vi "Generate Thetas.vi"(0 "spline flat":cluster{"x":sgl, "y":sgl}[](array[cluster]), 5 "starting angle":sgl, 7 "dt":sgl=0.02, 9 "ctrl pts":cluster{sgl, sgl}[][](array[cluster]), 11 "y unflat":cluster{dbl[]}[](array[cluster])) -> (4 "omega":sgl[](array[numeric]), 6 "theta":sgl[](array[numeric]), 10 "Tangent Vector":cluster{"x out":dbl, "y out":dbl}[](array[cluster]))   [LabVIEW 2025]
uses:
  <vilib>/Analysis/NI_AALPro.lvlib
panel:
  out "error":i32
  out "integral of P(x)":dbl
  out "Better omega":dbl(graph)
  out "Omega Theta":cluster{sgl, sgl}(graph)
  out "Array 2":sgl[](array[numeric])
  out "Array":sgl[](array[numeric])
  out "Thetas":sgl(graph)
  out "Omegas":sgl(graph)
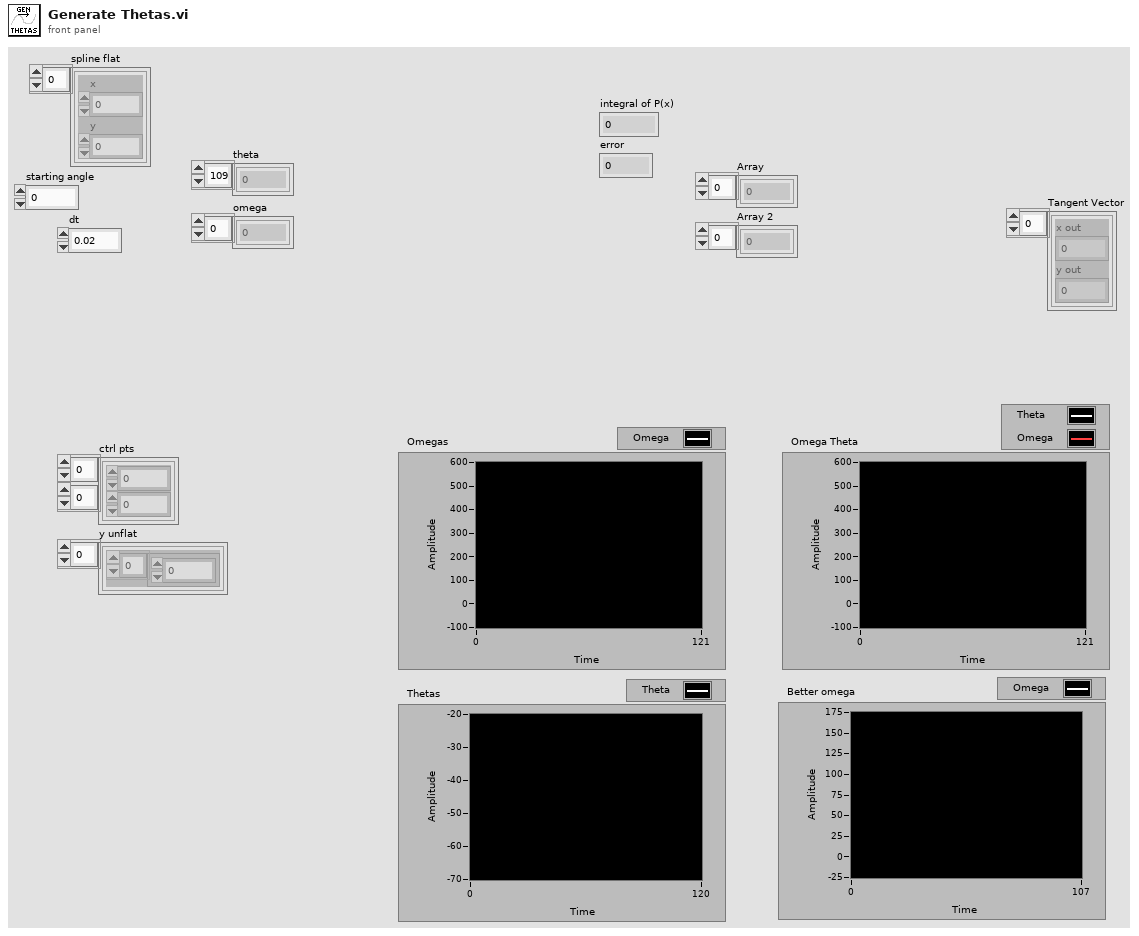
[diagram p1: front panel]
types:
  T1 = typedef "Bezier Curve.ctl" = cluster{"x":sgl, "y":sgl}[]
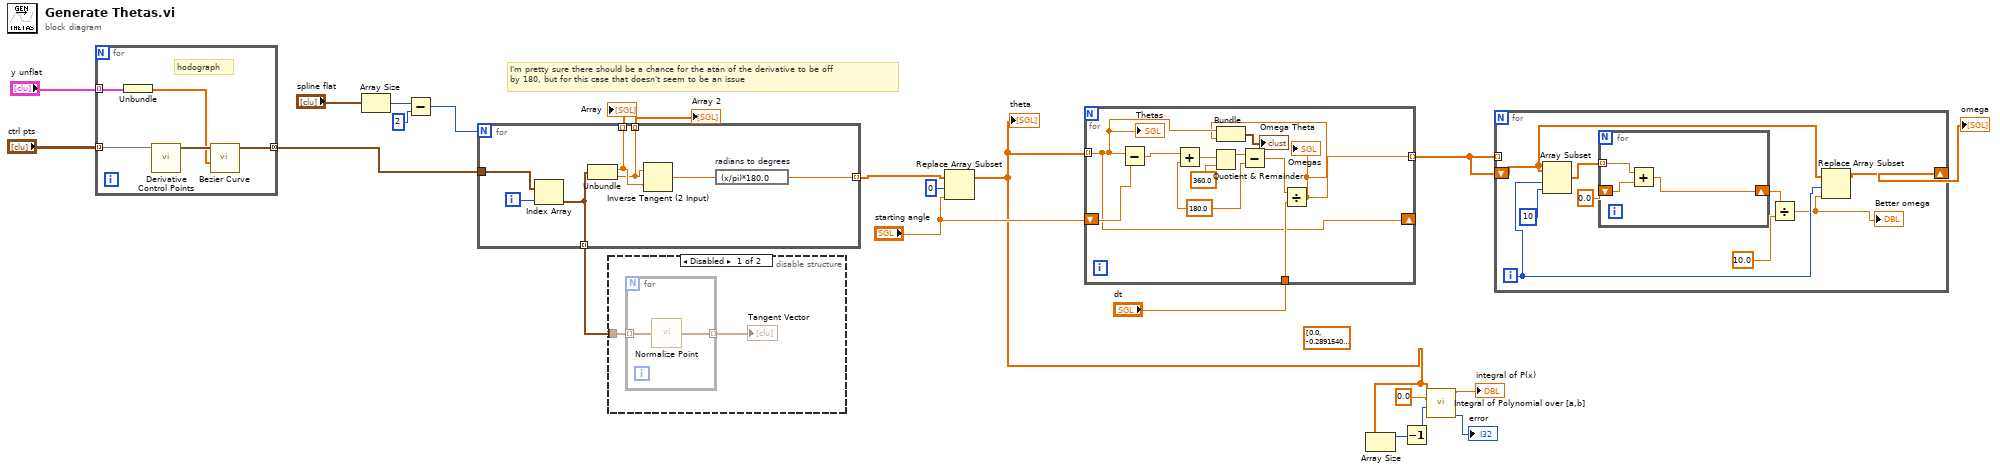
[diagram p0: block diagram]
diagram:
  (unwired) sgl[] [0.0, -0.28915405, -2.3239136, -4.3907166, -6.045532, -7.305908, -8.300018, -9.1796875, -10.028076, -10.773468, -11.160278, -10.85968, -9.686279, -7.7842712, -5.5885315, -3.5728455, -1.9668579, -0.58517456, 1.1642456, 3.9718628, 7.899475, 11.872864, 14.99176, 20.056915, 36.964417, 88.8649, 225.06256, 273.28796, 0.82702637, 0.0, 326.27335, 23.78769, -12.390137, 52.496338, 56.074524, 23.157501, 5.381012, -0.012207031, 3.9520264, 8.261108, 6.694031, 3.0174255, 0.6744385, 0.8544922, 2.4879456, 3.1822205, 2.3544312, 1.0757446, 0.4295349, 0.7759094, 1.5350342, 1.8356323, 1.4511108, 0.79345703, 0.41503906, 0.5645752, 1.0223389, 1.3381958, 1.2504578, 0.86517334, 0.50354004, 0.44174194, 0.692749, 1.0314941, 1.1886597, 1.0559082, 0.75302124, 0.51727295, 0.52337646, 0.75912476, 1.0482788, 1.1901855, 1.096344, 0.8514404, 0.64697266, 0.642395, 0.8468628, 1.1329651, 1.3206482, 1.3031006, 1.1146545, 0.91400146, 0.8682251, 1.0391235, 1.3381958, 1.6067505, 1.7036438, 1.6082764, 1.435852, 1.3633728, 1.5014648, 1.8295288, 2.2148132, 2.5032043, 2.6153564, 2.6000977, 2.607727, 2.7900696, 3.2234192, 3.8871765, 4.712677, 5.621338, 6.550598, 7.470703, 8.502197, 10.179901, 13.85498, 22.315979, 41.5596, 86.88583, 197.18704, 580.2109, 216.07513, 166.86935, 106.74896, 70.41855, 54.12903, 46.938324, 40.138245, 31.302643, 22.782898, 17.404175, 15.653229, 15.362549, 13.935852, 10.971069, 8.059692, 6.6085815, 6.3949585, 5.9906006, 4.634857, 3.0097961, 1.9348145, 1.3092041, 0.45776367, -0.75912476, -1.7349243, -2.3475647, -3.2951355, -4.974365, -6.7489624, -7.574463, -7.5180054, -7.8674316, -9.4314575, -11.539459, -12.7204895, -12.154388, -10.472107, -8.982849, -8.395386, -8.442688, -8.370972, -7.6019287, -6.1294556, -4.3884277, -2.8549194, -1.7570496, -1.0910034, -0.7522583, -0.62332153, -0.5996704, -0.5897522] ("Array 3")
  # "I'm pretty sure there should be a chance for the atan of the derivative to be off\nby 180, but for this case that doesn't seem to be an issue"
  n1 = for {
    tunnel: "ctrl pts" -> [w27] mode=indexing
    tunnel: "y unflat" -> [w25] mode=indexing
    tunnel: [w23] -> w15 mode=concatenating
    # "hodograph"
    n2 = Unbundle(w25) -> (w24:dbl[])
    n3 = call "Derivative Control Points.vi"("ctrl points"=w27) -> ("d ctrl pts"=w26:cluster{dbl, dbl}[])  [unwired: 10 in]
    n4 = call "Bezier Curve.vi"("position"=w24, "ctrl points"=w26) -> ("curve"=w23:T1)  [unwired: 8 in, 1 out]
  }
  n5 = Array Size(array="spline flat") -> (size(s)=w22:i32)
  n6 = Subtract(x=w22, y=2) -> (x-y=w20:i32)
  n7 = for {
    N: w20 -> [_]
    tunnel: w15 -> [w32]
    tunnel: [w33] -> w9 mode=indexing
    tunnel: [w30] -> w12 mode=indexing
    tunnel: [w29] -> w11 mode=indexing
    tunnel: [w28] -> w10 mode=indexing
    i -> [w31]
    n8 = Index Array(array=w32, index=w31) -> (element=w30:cluster{"x":sgl, "y":sgl})
    n9 = Unbundle(w30) -> ("x"=w29:sgl, "y"=w28:sgl)
    n10 = Inverse Tangent (2 Input)(1:w29, 2:w28) -> (0:w34:sgl)
    n11 = expression code="(x/pi)*180.0" "radians to degrees"(w34) -> (w33:sgl)
  }
  "Array" <- w11
  "Array 2" <- w10
  n12 = disable-structure shown="Disabled" {
    disable-tunnel: w12 -> [w36 _]
    frame Disabled {
      n13 = for {
        tunnel: w36 -> [w37] mode=indexing
        tunnel: [w38] -> w35 mode=indexing
        n14 = call "Normalize Point.vi"("point in"=w37) -> ("point out"=w38:cluster{"x":sgl, "y":sgl})
      }
      "Tangent Vector" <- w35
    }
    frame Enabled {
    }
  }
  n15 = Replace Array Subset(array=w9, new element="starting angle", index=0) -> (w1:sgl[])
  "theta" <- w1
  n16 = for {
    tunnel: w1 -> [w41] mode=indexing
    shift-right: [w41] -> _
    shift-left: "starting angle" -> [w49]
    tunnel: [w40] -> w2 mode=indexing
    tunnel: "dt" -> [w48]
    w42 = sgl 180.0 ("y")
    n17 = Subtract(x=w41, y=w49) -> (x-y=w47:sgl)
    n18 = Add(x=w47, y=w42) -> (x+y=w46:sgl)
    n19 = Quotient & Remainder(x=w46, y=sgl 360.0) -> (x-y*floor(x/y)=w43:sgl)  [unwired: 1 out]
    n20 = Subtract(x=w43, y=w42) -> (x-y=w44:sgl)
    n21 = Divide(x=w44, y=w48) -> (x/y=w40:sgl)
    "Omegas" <- w40
    n22 = Bundle(w41, w40) -> (→"Omega Theta":cluster{sgl, sgl})  [unwired: 1 in]
    "Thetas" <- w41
  }
  n23 = Array Size(array=w1) -> (size(s)=w3:i32)
  n24 = Decrement(x=w3) -> (x-1=w4:i32)
  n25 = call <vilib>:"Integral of Polynomial over [a,b].vi"("b"=w4, "a"=0.0, "P(x)"=w1) -> ("error"=→"error":i32, "integral of P(x)"=→"integral of P(x)":dbl)  [unwired: 7 in]
  n26 = for {
    tunnel: w2 -> [_] mode=indexing
    shift-right: [w50] -> w5
    shift-left: w2 -> [w53]
    i -> [w52]
    n27 = Array Subset(array=w53, index=w52, length=10) -> (w57:sgl[])
    n28 = for {
      tunnel: w57 -> [w60] mode=indexing
      shift-right: [w59] -> w55
      shift-left: 0.0 -> [w61]
      n29 = Add(x=w60, y=w61) -> (x+y=w59:dbl)
    }
    n30 = Divide(x=w55, y=10.0) -> (x/y=w51:dbl)
    "Better omega" <- w51
    n31 = Replace Array Subset(array=w53, new element=w51, index=w52) -> (w50:sgl[])
  }
  "omega" <- w5
